vi "MainGUI.vi"(8 "ErrorIn":errorcluster, 11 "OpenCVCamIn":refnum<class "OpenCVCam.lvclass">) -> ()   [LabVIEW 2021, in "OpenCVCam.lvclass"]
uses:
  OpenCVCam.lvclass
  C:/Localdata/Projects/TriekselSoft/TriekselsoftApplicationFramework/Source/.Externals/Library_YAF/YActor/YActor.lvclass
  OpenCVCam.lvclass/OpenCVCam.ctl
  OpenCVCam_UiCallBackEvents.ctl
  c1ad68ea-9d58-4aa5-81ea-12a966c9aacc.vi
  OpenCVCam_ClassCast.vi
  .Externals/Library_YAF/YActor/YActor.lvclass
  <vilib>/ptbypt/NI_PtbyPt.lvlib
panel:
  out "Framerate":dbl format="%0.0f Hz"
  out "State":string
  in  "Start":bool
  out "L_busy":i32
  out "Image":picture
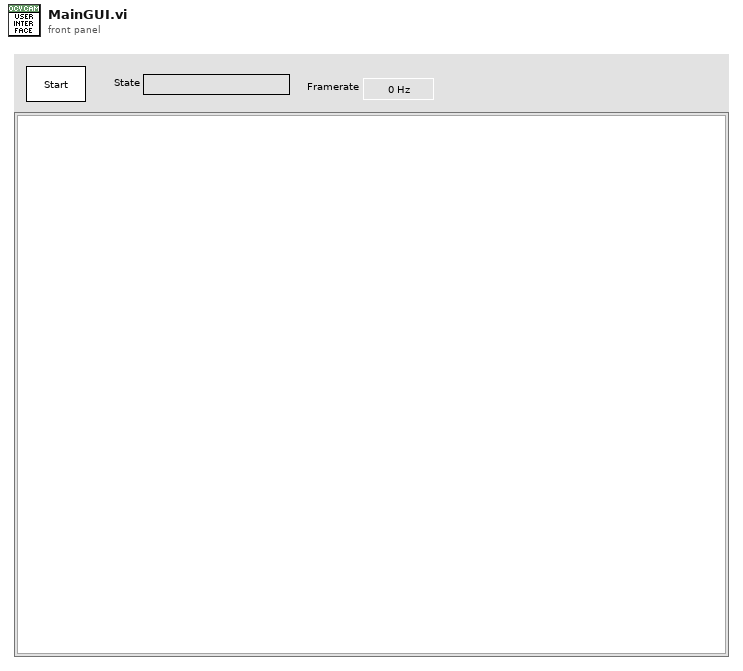
[diagram p1: front panel]
types:
  T1 = typedef "OpenCVCam.lvclass/OpenCVCam_UiCallBackEvents.ctl" = enum16{"Default", "PersistentDataUpdated", "NewPicture", "Worker 1: Do Something"}
  T2 = cluster{"Event":string, "This":refnum<class>, "Data":variant}
  T3 = typedef "imagedata.ctl" = cluster{"image type":i32, "image depth":i32, "image":u8[], "mask":u8[], "colors":u32[], "Rectangle":cluster{"left":i16, "top":i16, "right":i16, "bottom":i16}}
  T4 = typedef "OpenCVCam.lvclass/State.ctl" = enum16{"Idle", "Initialized", "Acquiring"}
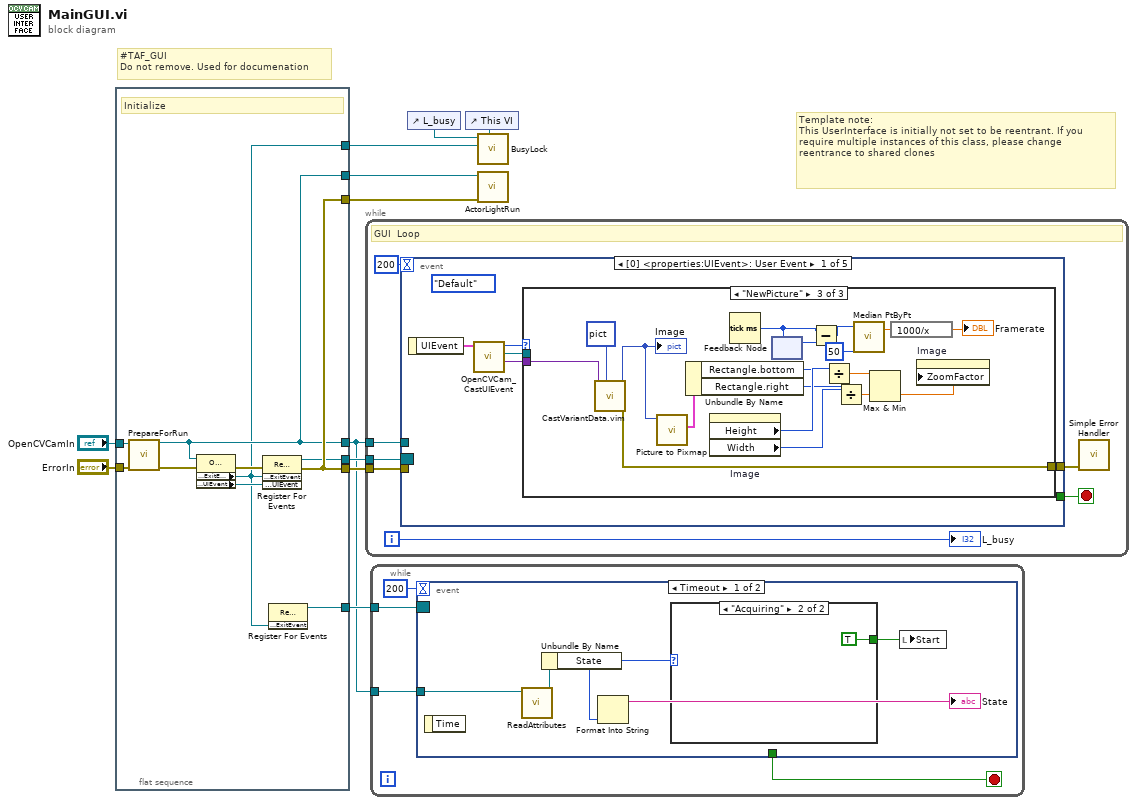
[diagram p0: block diagram]
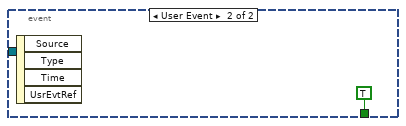
[diagram p3: hidden frame]
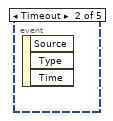
[diagram p6: hidden frame]
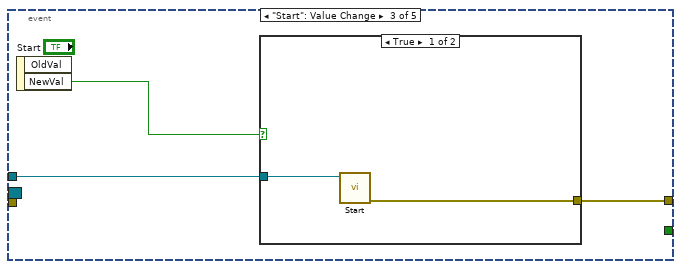
[diagram p7: hidden frame]
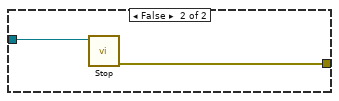
[diagram p8: hidden frame]
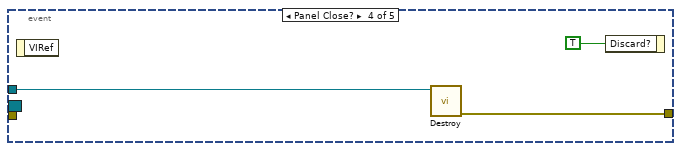
[diagram p9: hidden frame]
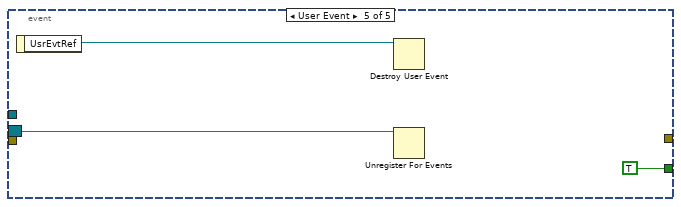
[diagram p10: hidden frame]
diagram:
  # "#TAF_GUI\nDo not remove. Used for documenation"
  # "Template note:\nThis UserInterface is initially not set to be reentrant. If you require multiple instances of this class, please change reentrance to shared clones"
  n1 = flat-sequence {
    tunnel: "ErrorIn" -> [w21]
    tunnel: "OpenCVCamIn" -> [w17]
    tunnel: [w16] -> w7
    tunnel: [w13] -> w4
    tunnel: [w15] -> w1
    tunnel: [w18] -> w10
    tunnel: [w15] -> w3
    tunnel: [w18] -> w9
    tunnel: [w12] -> w2
    frame #0 {
      # "Initialize"
      n2 = call-dynamic "PrepareForRun.vi"("ErrorIn"=w21, "YActorIn"=w17) -> ("ErrorOut"=w19:errorcluster, "YActorOut"=w15:refnum<class "OpenCVCam.lvclass">)  [unwired: 8 in]
      n3 = property class="OpenCVCam"(reference=w15, error in=w19) -> (error out=w20:errorcluster, "properties:ExitEvent"=w13:refnum<user-event>, "properties:UIEvent"=w14:refnum<user-event>)  [unwired: 1 out]
      n4 = register-events(error in=w20, w13, w14) -> (reference out=w16:refnum<event-registration>, error out=w18:errorcluster)  [unwired: 1 in]
      n5 = register-events(w13) -> (reference out=w12:refnum<event-registration>)  [unwired: 2 in, 1 out]
    }
  }
  n6 = while {
    tunnel: w10 -> [w28]
    tunnel: w7 -> [w25]
    tunnel: w1 -> [w22]
    i -> [w24]
    stop <- w26 stop-if-true
    # "GUI  Loop"
    n7 = event shown="[0] <properties:UIEvent>: User Event" {
      selector: w25 -> [_ _ _ _ w63]
      dyn-events: _ -> [_ _ _ _ _]
      timeout: 200 -> [_ _ _ _ _]
      tunnel: w28 -> [_ _ _ _ _]
      tunnel: [_ _ _ _ TRUE] -> w26
      tunnel: [w33 _ w54 w61 _] -> w27
      tunnel: w22 -> [_ _ w52 w59 _]
      event User Event {
        (unwired) OpenCVCam_UiCallBackEvents."Default" ("UiEventNames")
        n8 = event-data() -> ("UIEvent"=w32:T2)  [unwired: 1 in]
        n9 = call "OpenCVCam_CastUIEvent.vi"("UIEvent"=w32) -> ("Data"=w29:variant, "ApplicationGUIOut"=w30:refnum<class "OpenCVCam.lvclass">, "UiEventNames"=w31:T1)  [unwired: 8 in]
        n10 = case shown="\"NewPicture\"" w31 {
          tunnel: w30 -> [_ _ _]
          tunnel: w29 -> [_ _ w50]
          tunnel: [_ _ w51] -> w33
          frame Default {
          }
          frame "PersistentDataUpdated" {
            # "Use these events as callbacks from your actor to update the user interface controls. This way your actor will not enter the ui thread, and all UI actions are handled in this VI."
          }
          frame "NewPicture" {
            n11 = call "CastVariantData.vim"("Type"=picture data[5B] ("2D Picture"), "DataIn"=w50) -> ("ErrorOut"=w51:errorcluster, "DataOut"=w41:picture)  [unwired: 8 in]
            "Image" <- w41
            n12 = call <vilib>:"Picture to Pixmap.vi"("picture"=w41) -> ("image data"=w42:T3)  [unwired: 9 in, 1 out]
            n13 = Unbundle By Name(w42) -> ("Rectangle.bottom"=w43:i16, "Rectangle.right"=w44:i16)
            n14 = property on="Image" class="Pict"() -> ("Height"=w47:u32, "Width"=w48:u32)  [unwired: 2 in, 2 out]
            n15 = Tick Count (ms)() -> (millisecond timer value=w38:u32)
            n16 = feedback-in #1(w38) -> ()
            n17 = feedback #1() -> (w39:u32)  [unwired: 1 in]
            n18 = Subtract(x=w38, y=w39) -> (x-y=w37:u32)
            n19 = Divide(x=w47, y=w43) -> (x/y=w46:dbl)
            n20 = Divide(x=w48, y=w44) -> (x/y=w45:dbl)
            n21 = call <vilib>:"Median PtByPt.vi"("sample length"=50, "x"=w37) -> ("median"=w35:dbl)  [unwired: 2 in, 1 out]
            n22 = Max & Min(x=w46, y=w45) -> (min(x,y)=w40:dbl)  [unwired: 1 out]
            n23 = expression code="1000/x"(w35) -> (→"Framerate":dbl)
            n24 = property on="Image" class="Pict"("ZoomFactor"=w40) -> ()  [unwired: 2 in, 2 out]
          }
        }
      }
      event Timeout {
        n25 = event-data() -> ()  [unwired: 1 in, 3 out]
      }
      event "Start": Value Change {
        n26 = event-data() -> ("NewVal"=w53:bool)  [unwired: 1 in, 1 out]
        n27 = case shown="True" w53 {
          tunnel: w52 -> [w55 w57]
          tunnel: [w56 w58] -> w54
          frame True {
            n28 = call-dynamic "Start.vi"("OpenCVCamIn"=w55) -> ("ErrorOut"=w56:errorcluster)  [unwired: 9 in, 1 out]
          }
          frame False {
            n29 = call-dynamic "Stop.vi"("OpenCVCamIn"=w57) -> ("ErrorOut"=w58:errorcluster)  [unwired: 9 in, 1 out]
          }
        }
      }
      event Panel Close? {
        n30 = event-data() -> ()  [unwired: 1 in, 1 out]
        n31 = call-dynamic "Destroy.vi"("ObjectIn"=w59) -> ("ErrorOut"=w61:errorcluster)  [unwired: 9 in, 1 out]
        n32 = event-data("Discard?"=TRUE) -> ()  [unwired: 1 in, 1 out]
      }
      event User Event {
        n33 = event-data() -> ("UsrEvtRef"=w62:refnum<user-event>)  [unwired: 1 in]
        n34 = Destroy User Event(user event=w62) -> ()  [unwired: 1 in, 1 out]
        n35 = Unregister For Events(event registration refnum=w63) -> ()  [unwired: 1 in, 1 out]
      }
    }
    n36 = call <vilib>:"Simple Error Handler.vi"("error in (no error)"=w27) -> ()  [unwired: 4 in, 5 out]
    "L_busy" <- w24
  }
  n37 = while {
    tunnel: w2 -> [w68]
    tunnel: w1 -> [w65]
    stop <- w67 stop-if-true
    n38 = event shown="[0] Timeout" {
      selector: w68 -> [_ _]
      dyn-events: _ -> [_ _]
      timeout: 200 -> [_ _]
      tunnel: [_ TRUE] -> w67
      tunnel: w65 -> [w69 _]
      event Timeout {
        n39 = event-data() -> ()  [unwired: 1 in, 1 out]
        n40 = call "ReadAttributes.vi"("YActorIn"=w69) -> ("YActorOut"=w70:refnum<class "OpenCVCam.lvclass">)  [unwired: 9 in, 1 out]
        n41 = Unbundle By Name(w70) -> ("State"=w73:T4)
        n42 = Format Into String(w73) -> (resulting string=→"State":string)  [unwired: 3 in, 1 out]
        n43 = case shown="\"Acquiring\"" w73 {
          tunnel: [_ TRUE ("Start")] -> w71
          frame Default {
          }
          frame "Acquiring" {
          }
        }
        n44 = local write "Start"(w71) -> ()
      }
      event User Event {
        n45 = event-data() -> ()  [unwired: 1 in, 4 out]
      }
    }
  }
  n46 = control-ref of="L_busy"() -> (w6:refnum<vi>)
  n47 = control-ref of="This VI"() -> (w5:refnum<vi>)
  n48 = call "BusyLock.vi"("BusyLock"=w5, "ExitEvent"=w4, "Counter"=w6) -> ()  [unwired: 9 in]
  n49 = call "ActorLightRun.vi"("ErrorIn"=w9, "YActorIn"=w3) -> ()  [unwired: 8 in, 2 out]
